vi "loadNodeGlyph.vi"(7 "glyphArray":string[](array[string]), 8 "error in (no error)":errorcluster, 10 "TreeCtl* in":refnum<vi>, 11 "xceDataNode in":refnum<class "xceDataNode.lvclass">) -> (0 "error out":errorcluster, 2 "TreeCtl* out":refnum<vi>, 3 "xceDataNode out":refnum<class "xceDataNode.lvclass">)   [LabVIEW 2013, in "xceDataNode.lvclass"]
doc: "Finds the index of a glyph, and sets the glyph in the tree control for the particular node."
uses:
  xceDataNode.lvclass
  xceNode/xceNode.lvclass
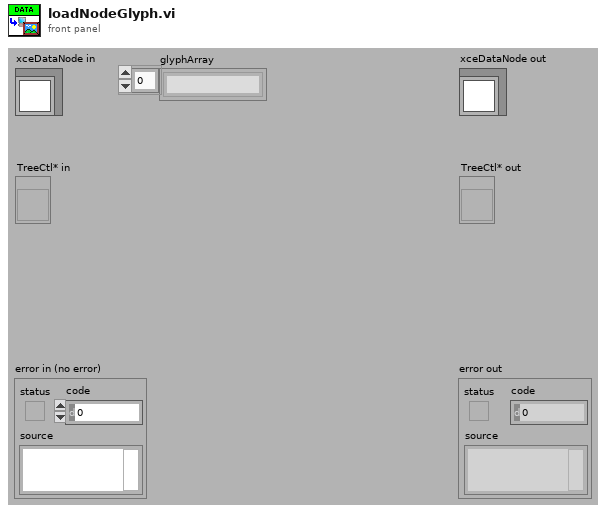
[diagram p1: front panel]
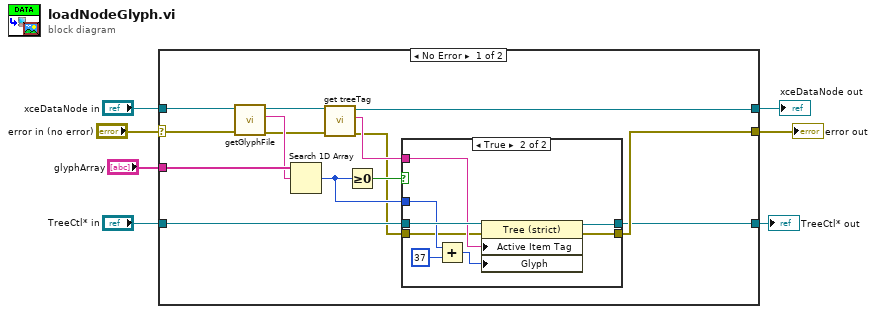
[diagram p0: block diagram]
diagram:
  n1 = case shown="No Error" "error in (no error)" {
    selector: "error in (no error)" -> [w12 w34]
    tunnel: [w9 w34] -> w6
    tunnel: [w13 w33] -> w4
    tunnel: "xceDataNode in" -> [w21 w33]
    tunnel: "TreeCtl* in" -> [w16 w32]
    tunnel: "glyphArray" -> [w20 _]
    tunnel: [w8 w32] -> w1
    frame No Error {
      n2 = call-dynamic "getGlyphFile.vi"("error in (no error)"=w12, "xceDataNode in"=w21) -> ("error out"=w11:errorcluster, "Glyph File"=w19:string, "xceDataNode out"=w15:refnum<class "xceDataNode.lvclass">)  [unwired: 7 in]
      n3 = Search 1D Array(1D array=w20, element=w19) -> (index of element=w17:i32)  [unwired: 1 in]
      n4 = call "get treeTag.vi"("error in (no error)"=w11, "xceNode in"=w15) -> ("error out"=w10:errorcluster, "treeTag"=w14:string, "xceNode out"=w13:refnum<class "xceDataNode.lvclass">)  [unwired: 7 in]
      n5 = Greater Or Equal To 0?(x=w17) -> (x >= 0?=w18:bool)
      n6 = case shown="True" w18 {
        tunnel: w17 -> [_ w28]
        tunnel: w16 -> [w22 w31]
        tunnel: w14 -> [_ w30]
        tunnel: w10 -> [w23 w26]
        tunnel: [w23 w25] -> w9
        tunnel: [w22 w24] -> w8
        frame False {
        }
        frame True {
          n7 = Add(x=w28, y=37) -> (x+y=w29:i32)
          n8 = property class="Tree (strict)"(reference=w31, error in=w26, "Active Item Tag"=w30, "Glyph"=w29) -> (reference out=w24:refnum<vi>, error out=w25:errorcluster)
        }
      }
    }
    frame Error {
    }
  }
  "error out" <- w6
  "xceDataNode out" <- w4
  "TreeCtl* out" <- w1
